vi "Other Wire Term.vi"(7 "Known Term":refnum<vi>, 10 "error in (no error)":errorcluster, 11 "Wire Terms":refnum<vi>[](array[refnum])) -> (2 "error out":errorcluster, 3 "Other Term":refnum<vi>)   [LabVIEW 2022 SP3, in "FlexBlocks Support.lvlib"]
uses:
  FlexBlocks Support.lvlib
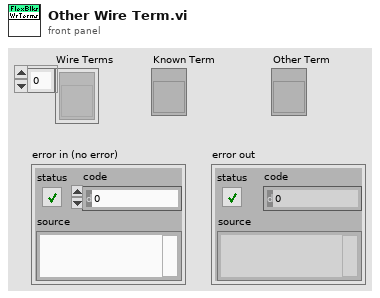
[diagram p1: front panel]
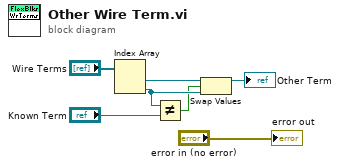
[diagram p0: block diagram]
diagram:
  n1 = Index Array(array="Wire Terms") -> (element #1=w6:refnum<vi>, element #2=w5:refnum<vi>)  [unwired: 2 in]
  n2 = Not Equal?(x=w5, y="Known Term") -> (x != y?=w4:bool)
  n3 = Swap Values(12:w6, 13:w4, 14:w5) -> (1:→"Other Term":refnum<vi>)  [unwired: 1 out]
  "error out" <- "error in (no error)"
